vi "Read Attributes.vi"(11 "new data number Msg":refnum<class "new data number Msg.lvclass">) -> (2 "Payload":cluster{"number":string})   [LabVIEW 2020, in "TouchScreen.lvlib" / "new data number Msg.lvclass"]
uses:
  new data number Msg.lvclass
  new data number Msg.lvclass/new data number Msg.ctl
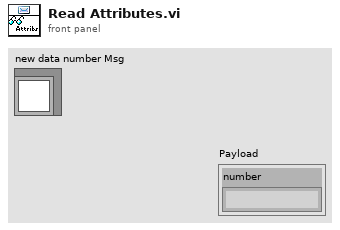
[diagram p1: front panel]
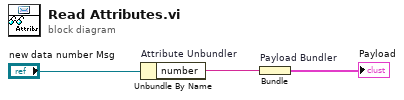
[diagram p0: block diagram]
diagram:
  n1 = Unbundle By Name "Attribute Unbundler"("new data number Msg") -> ("number"=w1:string)
  n2 = Bundle "Payload Bundler"("number"=w1) -> (→"Payload":cluster{"number":string})  [unwired: 1 in]
